vi "MaximizeWindow.vi"(8 "No Error":errorcluster, 11 "Window [SDL_Window *]":i64) -> (0 "Error Out":errorcluster)   [LabVIEW 2024, in "SDL3.lvlib" / "Video.lvlib"]
doc: "<B>Summary</B>\nRequest that the window be made as large as possible.\n\n<B>Remarks</B>\nNon-resizable windows can't be maximized. The window must have the <B>SDL_WINDOW_RESIZABLE</B> flag set, or this will have no effect.\n\nOn some windowing systems this request is asynchronous and the new window state may not have have been applied immediately upon the return of this function. If an immediate change is required, call <B>SDL_SyncWindow()</B> to block until the changes have taken effect.\n\nWhen the window state changes, an <B>SDL_EVENT_WINDOW_MAXIMIZED</B> event will be emitted. Note that, as this is just a request, the windowing system can deny the state change.\n\nWhen maximizing a window, whether the constraints set via <B>SDL_SetWindowMaximumSize()</B> are honored depends on the policy of the window manager. Win32 and macOS enforce the constraints when maximizing, while X11 and Wayland window managers may vary."
uses:
  Video.lvlib
  Error/Error.lvlib
  Lib/SDL3-32.dll
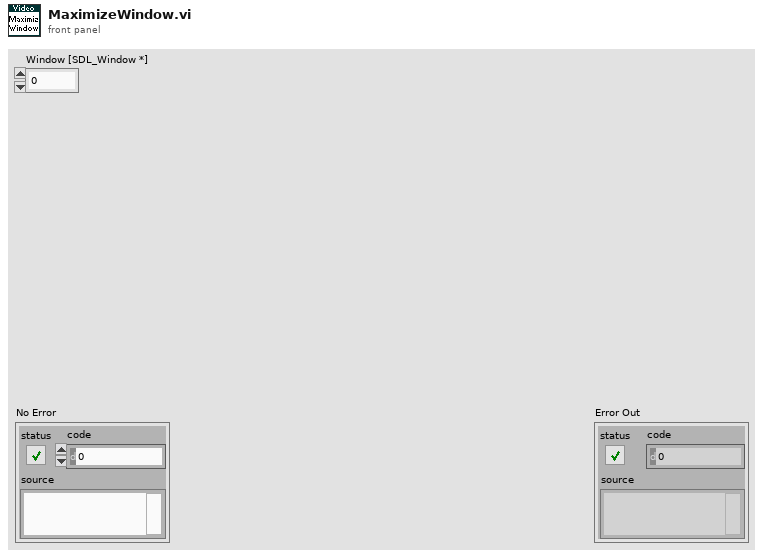
[diagram p1: front panel]
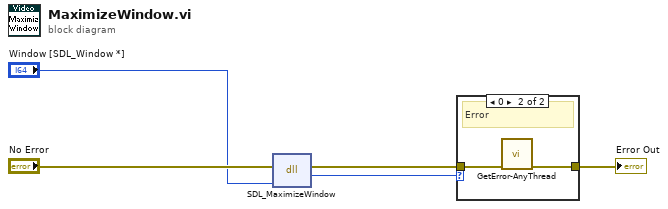
[diagram p0: block diagram]
diagram:
  n1 = dll-call lib="C:/Users/Thomas/Documents/Projects/LV-SDL3/Lib/SDL3-*.*" fn="SDL_MaximizeWindow"(error in="No Error", "window"="Window [SDL_Window *]") -> (error out=w3:errorcluster, "return type"=w1:i32)  [unwired: 3 in, 1 out]
  n2 = case shown="0" w1 {
    tunnel: w3 -> [w6 w8]
    tunnel: [w6 w7] -> w2
    frame Default {
      # "Ok"
    }
    frame 0 {
      # "Error"
      n3 = call "GetError-AnyThread.vi"("No Error"=w8) -> ("Error Out"=w7:errorcluster)  [unwired: 10 in]
    }
  }
  "Error Out" <- w2
